vi "GetChannelProbeAttenuation.vi"(8 "error in (no error)":errorcluster, 11 "TektronixDPO_PhysicalDevice.lvclass":refnum<class "TektronixDPO_PhysicalDevice.lvclass">) -> (0 "error out":errorcluster, 3 "TektronixDPO_PhysicalDevice.lvclassOut":refnum<class "TektronixDPO_PhysicalDevice.lvclass">)   [LabVIEW 2013, in "TektronixDPO_PhysicalDevice.lvclass"]
doc: "Read from the phsyical device the offset relative to the specified channel"
uses:
  TektronixDPO_PhysicalDevice.lvclass
  TektronixDPO_PhysicalDevice.lvclass/TektronixDPO_PhysicalDevice.ctl
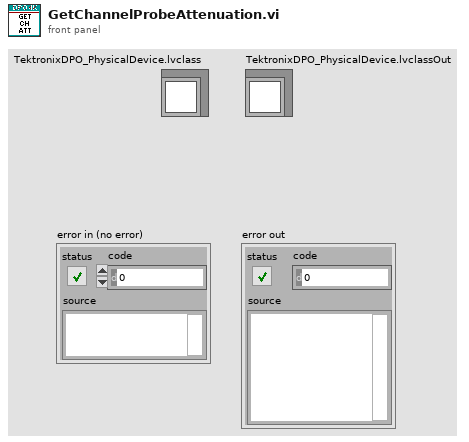
[diagram p1: front panel]
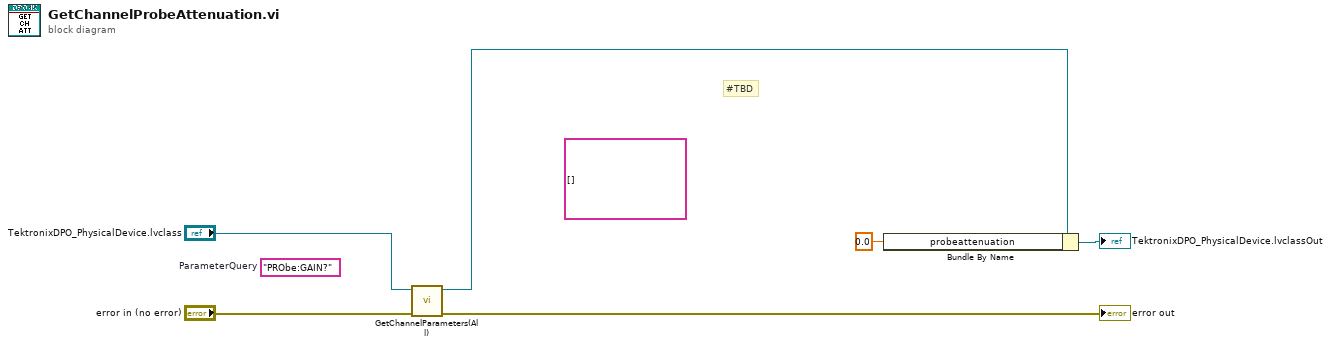
[diagram p0: block diagram]
diagram:
  (unwired) string[] [] ("1D array")
  (unwired) "PRObe:GAIN?"  # ParameterQuery
  # "#TBD"
  n1 = call "GetChannelParameters(All).vi"("error in (no error)"="error in (no error)", "TektronixDPO_PhysicalDevice in"="TektronixDPO_PhysicalDevice.lvclass") -> ("error out"=→"error out":errorcluster, "TektronixDPO_PhysicalDevice out"=w2:refnum<class "TektronixDPO_PhysicalDevice.lvclass">)  [unwired: 7 in, 1 out]
  n2 = Bundle By Name(cluster=w2, "probeattenuation"=0.0 ("ActiveChannel.Probe Attenuation")) -> (→"TektronixDPO_PhysicalDevice.lvclassOut":refnum<class "TektronixDPO_PhysicalDevice.lvclass">)
